vi "Query Questionable Status Register.vi"(8 "error in (no error)":errorcluster, 11 "VISA resource name":refnum<visa-resource-name>) -> (0 "error out":errorcluster, 2 "Questionable Status Register Value":u32, 3 "VISA resource name out":refnum<visa-resource-name>)   [LabVIEW 2022 SP3, in "MagnaDC.lvlib"]
uses:
  MagnaDC.lvlib
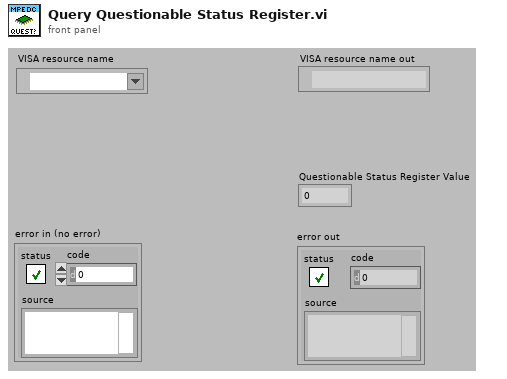
[diagram p1: front panel]
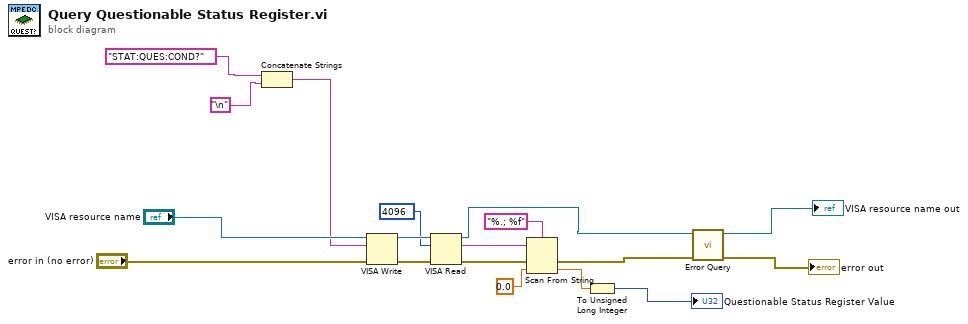
[diagram p0: block diagram]
diagram:
  n1 = Concatenate Strings("STAT:QUES:COND?" ("write buffer"), "\n") -> (w1:string)
  n2 = VISA Write(VISA resource name="VISA resource name", write buffer=w1, error in (no error)="error in (no error)") -> (VISA resource name out=w16:refnum<visa-resource-name>, error out=w15:errorcluster)  [unwired: 1 out]
  n3 = VISA Read(VISA resource name=w16, byte count=u32 4096, error in (no error)=w15) -> (VISA resource name out=w8:refnum<visa-resource-name>, read buffer=w13:string, error out=w11:errorcluster)  [unwired: 1 out]
  n4 = Scan From String(format string="%.; %f", input string=w13, error in=w11, default 1=0.0 ("default value 1")) -> (error out=w7:errorcluster, output 1=w9:dbl)  [unwired: 1 in, 2 out]
  n5 = To Unsigned Long Integer(number=w9) -> (unsigned 32bit integer=→"Questionable Status Register Value":u32)
  n6 = call "Error Query.vi"("error in (no error)"=w7, "VISA resource name"=w8) -> ("error out"=→"error out":errorcluster, "VISA resource name out"=→"VISA resource name out":refnum<visa-resource-name>)  [unwired: 6 in, 2 out]
